vi "FTW-JSON-LexicalScan-Error.vi"(0 "JSON String":T1, 7 "Error String":string, 11 "error in":errorcluster) -> (4 "JSON String Out":T1, 15 "error out":errorcluster)   [LabVIEW 2015]
uses:
  FTW-JSON-LexicalScan.ctl
panel:
  # "Inputs"
  # "Outputs"
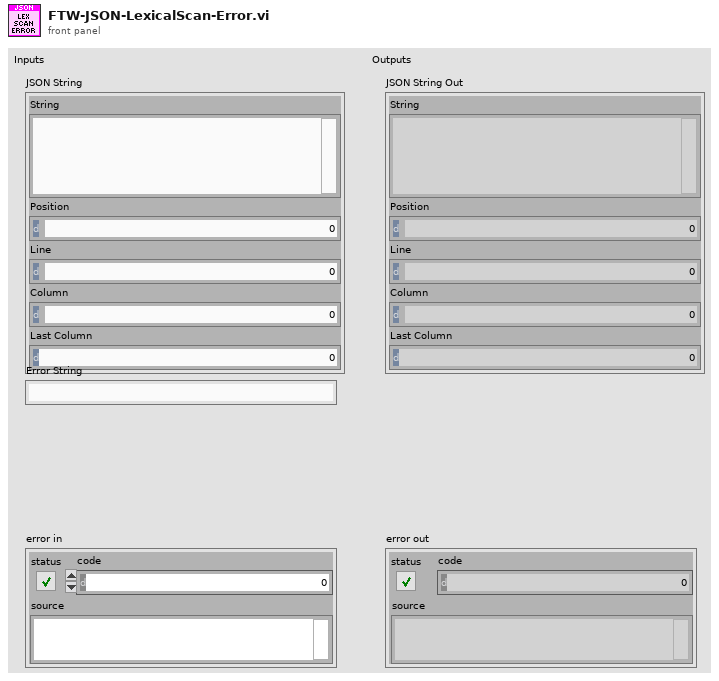
[diagram p1: front panel]
types:
  T1 = typedef "FTW-JSON-LexicalScan.ctl" = cluster{"String":string, "Position":i32, "Line":i32, "Column":i32, "Last Column":i32}
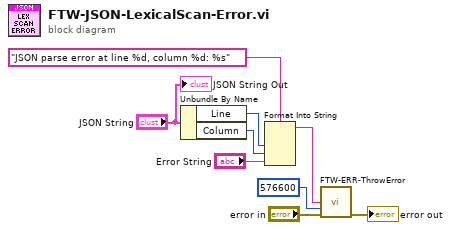
[diagram p0: block diagram]
diagram:
  n1 = Unbundle By Name("JSON String") -> ("Line"=w3:i32, "Column"=w2:i32)
  n2 = Format Into String(format string="JSON parse error at line %d, column %d: %s", w3, w2, "Error String") -> (resulting string=w5:string)  [unwired: 2 in, 1 out]
  n3 = call "FTW-ERR-ThrowError.vi"("Error Message"=w5, "Error Code"=576600, "error in"="error in") -> ("error out"=→"error out":errorcluster)  [unwired: 12 in]
  "JSON String Out" <- "JSON String"
